vi "BRig_dataMTrig_SolenoidCal_I_L.vi"() -> (2 "output_SolenoidCal_I_L":i32)   [LabVIEW 2014]
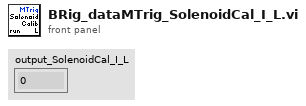
[diagram p1: front panel]
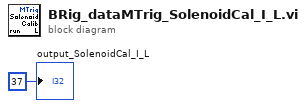
[diagram p0: block diagram]
diagram:
  "output_SolenoidCal_I_L" <- 37 ("output_iBlock")
